vi "Write Sub Panel prod.vi"(8 "error in (no error)":errorcluster, 10 "Sub Panel prod":refnum<vi>, 11 "coffe actor in":refnum<class "coffe actor.lvclass">) -> (0 "error out":errorcluster, 3 "coffe actor out":refnum<class "coffe actor.lvclass">)   [LabVIEW 2020, in "coffe actor.lvlib" / "coffe actor.lvclass"]
uses:
  coffe actor.lvclass
  coffe actor.lvclass/coffe actor.ctl
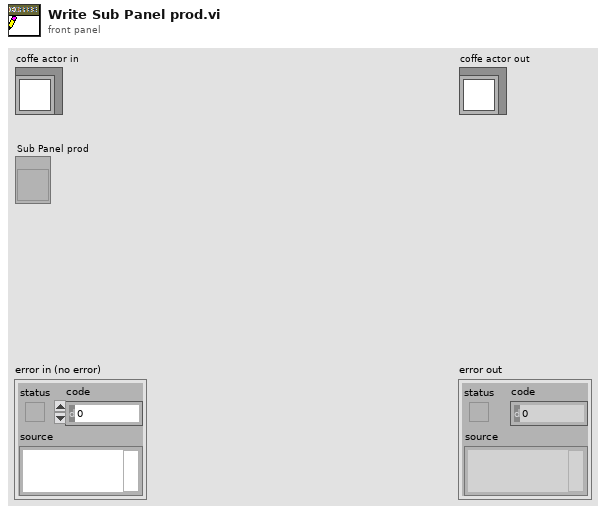
[diagram p1: front panel]
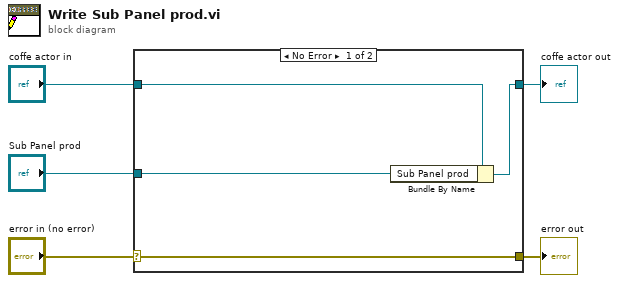
[diagram p0: block diagram]
diagram:
  n1 = case shown="No Error" "error in (no error)" {
    selector: "error in (no error)" -> [w9 w10]
    tunnel: [w9 w10] -> w4
    tunnel: [w7 w11] -> w2
    tunnel: "coffe actor in" -> [w8 w11]
    tunnel: "Sub Panel prod" -> [w6 _]
    frame No Error {
      n2 = Bundle By Name(cluster=w8, "Sub Panel prod"=w6) -> (w7:refnum<class "coffe actor.lvclass">)
    }
    frame Error {
    }
  }
  "error out" <- w4
  "coffe actor out" <- w2
